vi "oa_OrderResolution to BlockSize Enhanced.vi"(8 "error in (no error)":errorcluster, 10 "Order resolution (order)":dbl=0.1 min=0.0, 11 "Max order to analyze":dbl=64.0 format="%.2f") -> (0 "error out":errorcluster, 3 "Block size":i32)   [LabVIEW 2017]
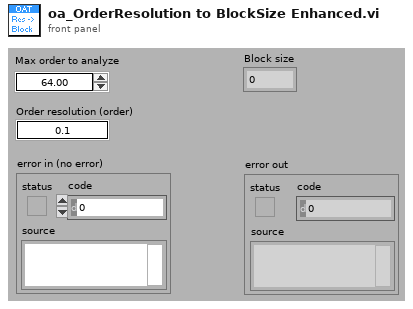
[diagram p1: front panel]
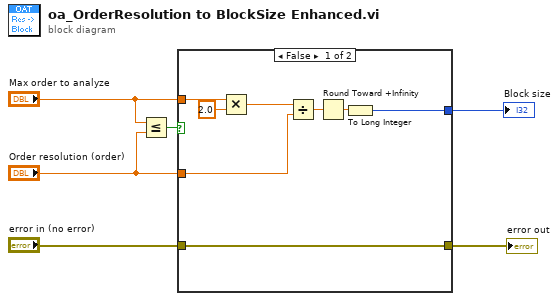
[diagram p0: block diagram]
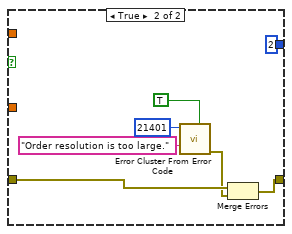
[diagram p2: hidden frame]
diagram:
  n1 = Less Or Equal?(x="Max order to analyze", y="Order resolution (order)") -> (x <= y?=w5:bool)
  n2 = case shown="False" w5 {
    tunnel: "Order resolution (order)" -> [w12 _]
    tunnel: "Max order to analyze" -> [w7 _]
    tunnel: [w11 2] -> w4
    tunnel: "error in (no error)" -> [w10 w17]
    tunnel: [w10 w15] -> w2
    frame False {
      n3 = Multiply(x=w7, y=2.0) -> (x*y=w8:dbl)
      n4 = Divide(x=w8, y=w12) -> (x/y=w14:dbl)
      n5 = Round Toward +Infinity(x=w14) -> (ceil(x): smallest int >= x=w13:dbl)
      n6 = To Long Integer(number=w13) -> (32bit integer=w11:i32)
    }
    frame True {
      n7 = call <vilib>:"Error Cluster From Error Code.vi"("is warning? (False)"=TRUE, "error message (\"\")"="Order resolution is too large." ("error message (\"\")"), "error code (0)"=21401) -> ("error out"=w16:errorcluster)  [unwired: 6 in]
      n8 = Merge Errors(w17, w16) -> (w15:errorcluster)
    }
  }
  "error out" <- w2
  "Block size" <- w4
